vi "CalSet_DirList.vi"(8 "error in (no error)":errorcluster, 11 "NetA_AgNA in":refnum<class "NetA_AgNA.lvclass">) -> (0 "error out":errorcluster, 1 "Cal Set Count":i32, 2 "Cal Set List":string[](array[string]), 3 "NetA_AgNA out":refnum<class "NetA_AgNA.lvclass">, 4 "Raw Dir List":string)   [LabVIEW 2014, in "NetA_AgNA.lvclass"]
doc: "Returns a list of the non-proprietary cal sets (located outside of the Keysight folders)."
uses:
  NetA_AgNA.lvclass
  NetA_AgNA.lvclass/NetA_AgNA.ctl
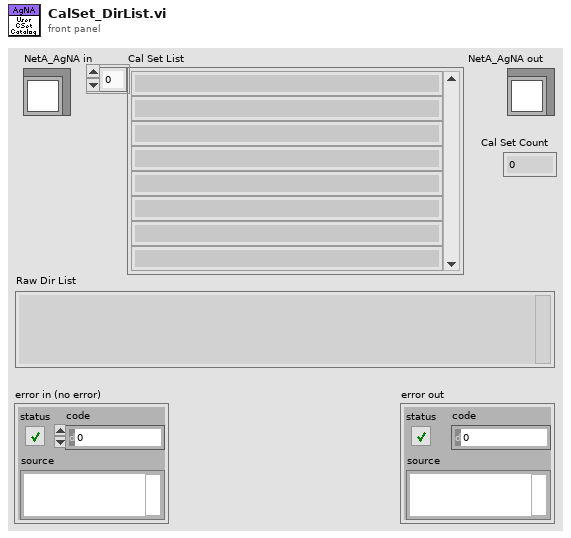
[diagram p1: front panel]
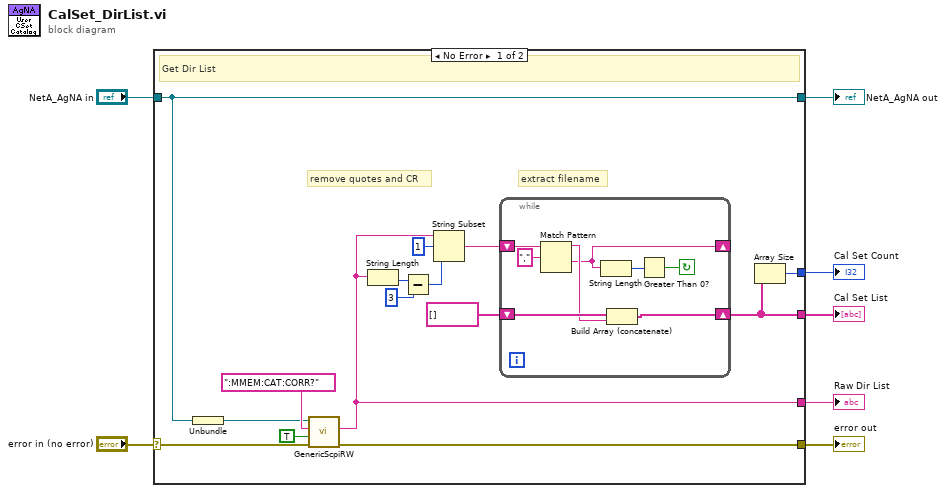
[diagram p0: block diagram]
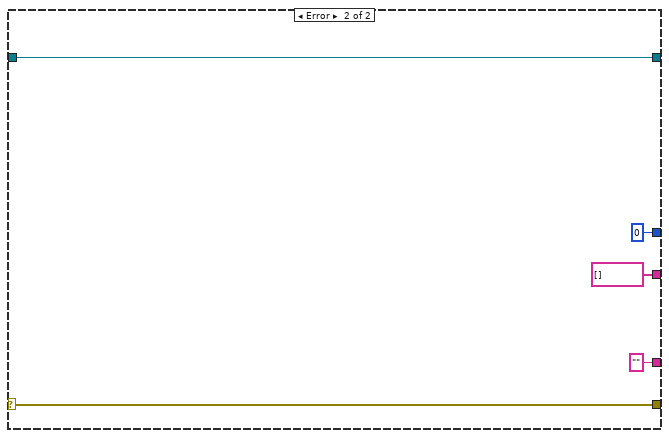
[diagram p2: hidden frame]
diagram:
  n1 = case shown="No Error" "error in (no error)" {
    selector: "error in (no error)" -> [w21 w34]
    tunnel: [w22 w34] -> w7
    tunnel: [w17 "" ("SCPI Response")] -> w5
    tunnel: [w11 string[] []] -> w4
    tunnel: [w10 0] -> w3
    tunnel: "NetA_AgNA in" -> [w9 w35]
    tunnel: [w9 w35] -> w1
    frame No Error {
      # "extract filename"
      # "remove quotes and CR"
      # "Get Dir List"
      n2 = Unbundle(w9) -> (w8:refnum<k15>)
      n3 = call "GenericScpiRW.vi"("error in (no error)"=w21, "Query?"=TRUE, "SCPI Command"=":MMEM:CAT:CORR?", "resource name"=w8) -> ("error out"=w22:errorcluster, "SCPI Response"=w17:string)  [unwired: 6 in]
      n4 = String Length(string=w17) -> (length=w16:i32)
      n5 = Subtract(x=w16, y=3) -> (x-y=w14:i32)
      n6 = String Subset(string=w17, offset (0)=1, length (rest)=w14) -> (substring=w12:string)
      n7 = while {
        shift-right: [w30] -> w11
        shift-left: string[] [] -> [w29]
        shift-right: [w25] -> _
        shift-left: w12 -> [w27]
        stop <- w23 continue-if-true
        n8 = Match Pattern(string=w27, regular expression=",") -> (before substring=w26:string, after substring=w25:string)  [unwired: 1 in, 2 out]
        n9 = String Length(string=w25) -> (length=w24:i32)
        n10 = Build Array (concatenate)(w29, w26) -> (w30:string[])
        n11 = Greater Than 0?(x=w24) -> (x > 0?=w23:bool)
      }
      n12 = Array Size(array=w11) -> (size(s)=w10:i32)
    }
    frame Error {
    }
  }
  "Raw Dir List" <- w5
  "error out" <- w7
  "Cal Set List" <- w4
  "Cal Set Count" <- w3
  "NetA_AgNA out" <- w1
